vi "Robot Global Data.vi"() -> ()   [LabVIEW 2011]
doc: "This global VI can contain as many global variables as you need. Place a control on the panel, give it a good name. To read or write to it from a VI, drag the icon to the diagram of that VI. You can also drag from the project. Click on the node to change which global you access. You shouldn't have multiple locations writing to a global or it will cause a race-condition."
uses:
  <vilib>/Rock Robotics/WPI/Camera/WPI_CameraImageSize.ctl
  Position Typedef.ctl
  Target Typedef.ctl
  Autonomous Data.ctl
  CAN Data.ctl
  ControlModes.ctl
  InitCounts.ctl
  ShooterData.ctl
panel:
  out "Shooter Data":T1
  out "Init Counts":T2
  in  "Use Camera":bool
  out "Shooter Mode":T3=enum."Key"
  out "Vision":T4
  in  "CAN Data":T5
  in  "Autonomous Data":T6
  out "Target":T7
  out "Position Data":T8
  in  "LED toggle rate (ms)":u32=20
  in  "image size":T9
  in  "Enable Vision":bool=TRUE
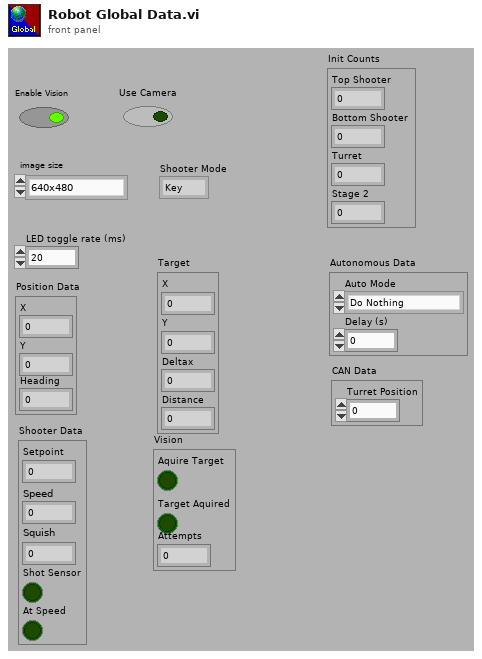
[diagram p1: front panel]
types:
  T1 = typedef "ShooterData.ctl" = cluster{"Setpoint":dbl, "Speed":dbl, "Squish":dbl, "Shot Sensor":bool, "At Speed":bool}
  T2 = typedef "InitCounts.ctl" = cluster{"Top Shooter":i8, "Bottom Shooter ":i8, "Turret":i8, "Stage 2":i8}
  T3 = typedef "ControlModes.ctl" = enum16{"Auto", "Key", "Fender", "Clearing"}
  T4 = cluster{"Aquire Target":bool, "Target Aquired":bool, "Attempts":dbl}
  T5 = typedef "CAN Data.ctl" = cluster{"Turret Position":dbl}
  T6 = typedef "Autonomous Data.ctl" = cluster{"Auto Mode":enum16{"Do Nothing", "Shoot From Key", "Shoot From Key Center, Bridge", "Shoot From Key, Feed", "Shoot From Key, Drive Forward", "Fender From Center", "Fender From Right", "Fender From Left"}, "Delay (s)":dbl}
  T7 = typedef "Target Typedef.ctl" = cluster{"X":dbl, "Y":dbl, "Deltax":dbl, "Distance":dbl}
  T8 = typedef "Position Typedef.ctl" = cluster{"X":dbl, "Y":dbl, "Heading":dbl}
  T9 = typedef "WPI_CameraImageSize.ctl" = enum16{"640x480", "320x240", "160x120"}
diagram:
